vi "ImageFileHeaderSubVI.vi"(0 "size x":i16, 1 "size y":i16, 2 "frame rate":i16, 3 "bin duration":i16, 4 "recording duration":u16) -> (7 "refnum out":refnum<file>)   [LabVIEW 2009]
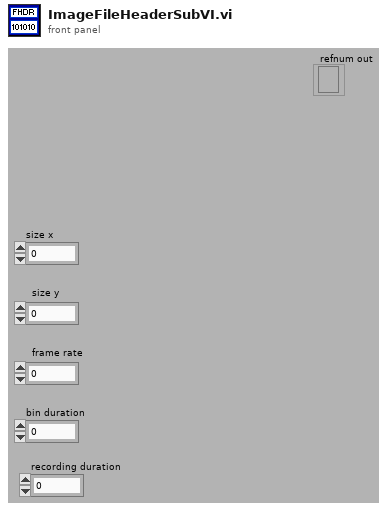
[diagram p1: front panel]
types:
  T1 = enum16{"open", "replace", "create", "open or create", "replace or create", "replace or create with confirmation"}
  T2 = enum16{"big-endian, network order", "native, host order", "little-endian"}
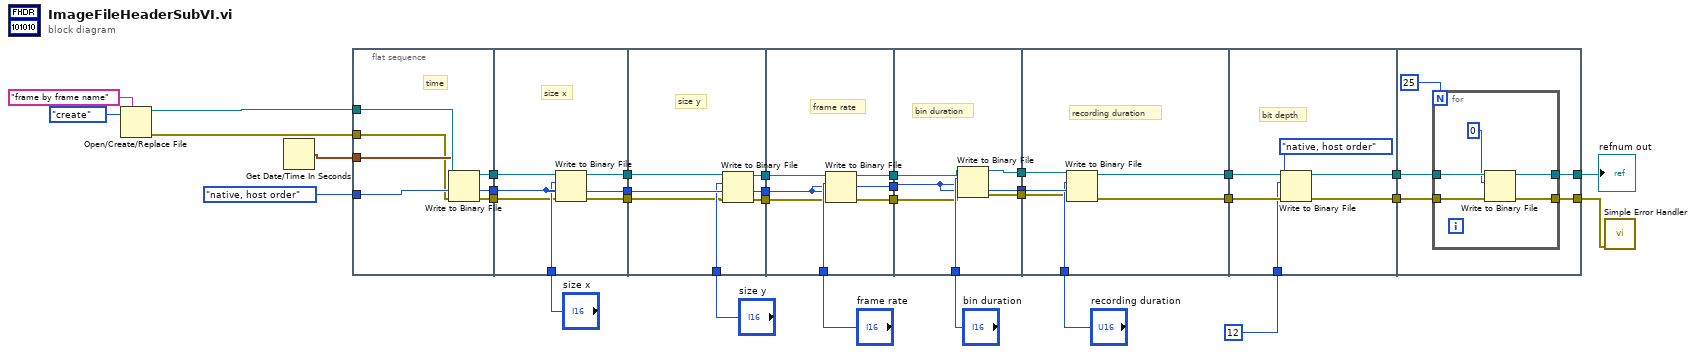
[diagram p0: block diagram]
diagram:
  n1 = Open/Create/Replace File(prompt="frame by frame name", operation (0:open)=T1."create") -> (refnum out=w17:refnum<file>, error out=w13:errorcluster)  [unwired: 4 in, 1 out]
  n2 = Get Date/Time In Seconds() -> (seconds since 1Jan1904=w20:timestamp)
  n3 = flat-sequence {
    tunnel: w17 -> [w39]
    tunnel: w20 -> [w38]
    tunnel: T2."native, host order" ("byte order (0:big-endian, network order)") -> [w36]
    tunnel: [w37] -> w33
    tunnel: [w36] -> w32
    tunnel: w13 -> [w35]
    tunnel: [w34] -> w12
    tunnel: w33 -> [w45]
    tunnel: w32 -> [w43]
    tunnel: [w44] -> w31
    tunnel: [w43] -> w30
    tunnel: "size x" -> [w42]
    tunnel: w12 -> [w41]
    tunnel: [w40] -> w11
    tunnel: w31 -> [w48]
    tunnel: w30 -> [w50]
    tunnel: [w50] -> w29
    tunnel: [w51] -> w28
    tunnel: "size y" -> [w49]
    tunnel: w11 -> [w47]
    tunnel: [w46] -> w10
    tunnel: w29 -> [w54]
    tunnel: w28 -> [w57]
    tunnel: "frame rate" -> [w56]
    tunnel: [w55] -> w27
    tunnel: [w54] -> w26
    tunnel: w10 -> [w53]
    tunnel: [w52] -> w9
    tunnel: w27 -> [w63]
    tunnel: w26 -> [w60]
    tunnel: "bin duration" -> [w62]
    tunnel: [w61] -> w16
    tunnel: [w60] -> w15
    tunnel: w9 -> [w59]
    tunnel: [w58] -> w8
    tunnel: w16 -> [w69]
    tunnel: w15 -> [w67]
    tunnel: "recording duration" -> [w66]
    tunnel: [w68] -> w7
    tunnel: w8 -> [w65]
    tunnel: [w64] -> w6
    tunnel: w7 -> [w75]
    tunnel: w6 -> [w74]
    tunnel: i16 12 ("bit depth") -> [w73]
    tunnel: [w72] -> w4
    tunnel: [w71] -> w3
    tunnel: w4 -> [w78]
    tunnel: w3 -> [w79]
    tunnel: [w77] -> w2
    tunnel: [w76] -> w1
    frame #0 {
      # "time"
      n4 = Write to Binary File(file (use dialog)=w39, data=w38, error in=w35, 9:w36) -> (refnum out=w37:refnum<file>, error out=w34:errorcluster)  [unwired: 2 in, 1 out]
    }
    frame #1 {
      # "size x"
      n5 = Write to Binary File(file (use dialog)=w45, data=w42, error in=w41, 9:w43) -> (refnum out=w44:refnum<file>, error out=w40:errorcluster)  [unwired: 2 in, 1 out]
    }
    frame #2 {
      # "size y"
      n6 = Write to Binary File(file (use dialog)=w48, data=w49, error in=w47, 9:w50) -> (refnum out=w51:refnum<file>, error out=w46:errorcluster)  [unwired: 2 in, 1 out]
    }
    frame #3 {
      # "frame rate"
      n7 = Write to Binary File(file (use dialog)=w57, data=w56, error in=w53, 9:w54) -> (refnum out=w55:refnum<file>, error out=w52:errorcluster)  [unwired: 2 in, 1 out]
    }
    frame #4 {
      # "bin duration"
      n8 = Write to Binary File(file (use dialog)=w63, data=w62, error in=w59, 9:w60) -> (refnum out=w61:refnum<file>, error out=w58:errorcluster)  [unwired: 2 in, 1 out]
    }
    frame #5 {
      # "recording duration"
      n9 = Write to Binary File(file (use dialog)=w69, data=w66, error in=w65, 9:w67) -> (refnum out=w68:refnum<file>, error out=w64:errorcluster)  [unwired: 2 in, 1 out]
    }
    frame #6 {
      # "bit depth"
      n10 = Write to Binary File(file (use dialog)=w75, data=w73, error in=w74, 9:T2."native, host order" ("byte order (0:big-endian, network order)")) -> (refnum out=w72:refnum<file>, error out=w71:errorcluster)  [unwired: 2 in, 1 out]
    }
    frame #7 {
      n11 = for {
        N: i64 25 ("offset (in bytes) (0)") -> [_]
        tunnel: w79 -> [w85]
        tunnel: w78 -> [w84]
        tunnel: [w83] -> w77
        tunnel: [w82] -> w76
        n12 = Write to Binary File(file (use dialog)=w84, data=i8 0, error in=w85) -> (refnum out=w83:refnum<file>, error out=w82:errorcluster)  [unwired: 3 in, 1 out]
      }
    }
  }
  n13 = call <vilib>:"Simple Error Handler.vi"("error in (no error)"=w1) -> ()  [unwired: 4 in, 5 out]
  "refnum out" <- w2
